vi "TrioMotion_Test.vi"() -> ()   [LabVIEW 2020]
panel:
  out "Error Out":errorcluster
  in  "stop":bool
  in  "Set Parameters":bool
  out "CommPort":fxp<+,3,3>
  in  "Open/ Close":bool
  in  "Connection":string(combo)
  out "IsOpen":bool
  in  "Error In (no error)":errorcluster
  in  "Connection":refnum<k7>(container)
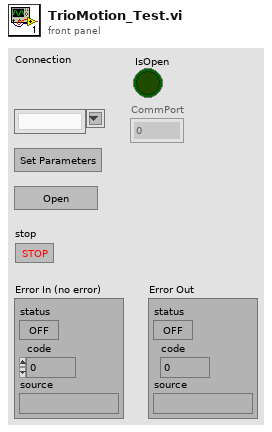
[diagram p1: front panel]
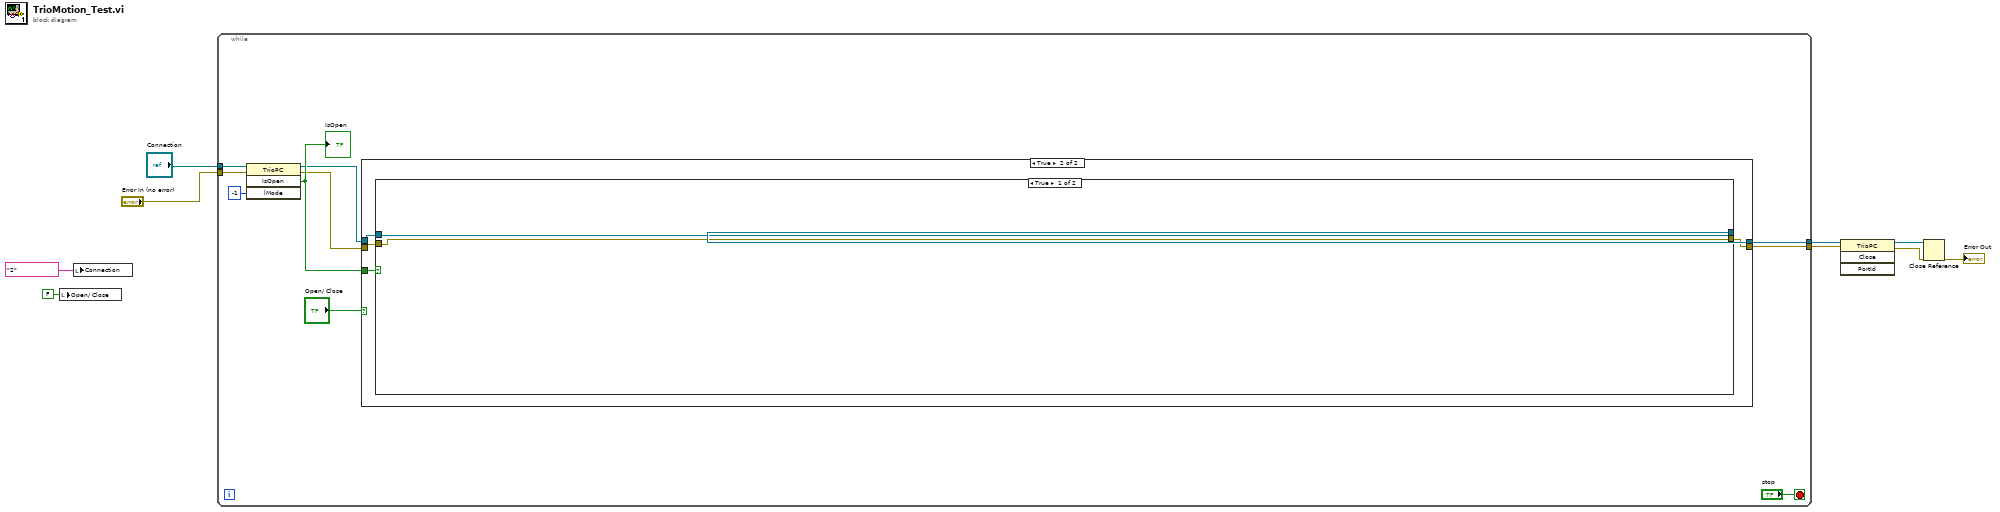
[diagram p0: block diagram]
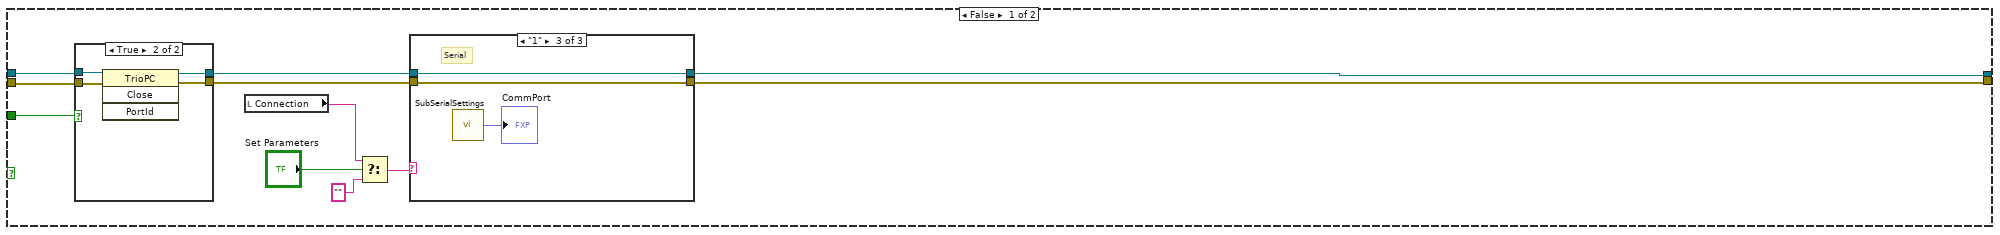
[diagram p2: hidden frame]
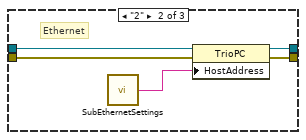
[diagram p4: hidden frame]
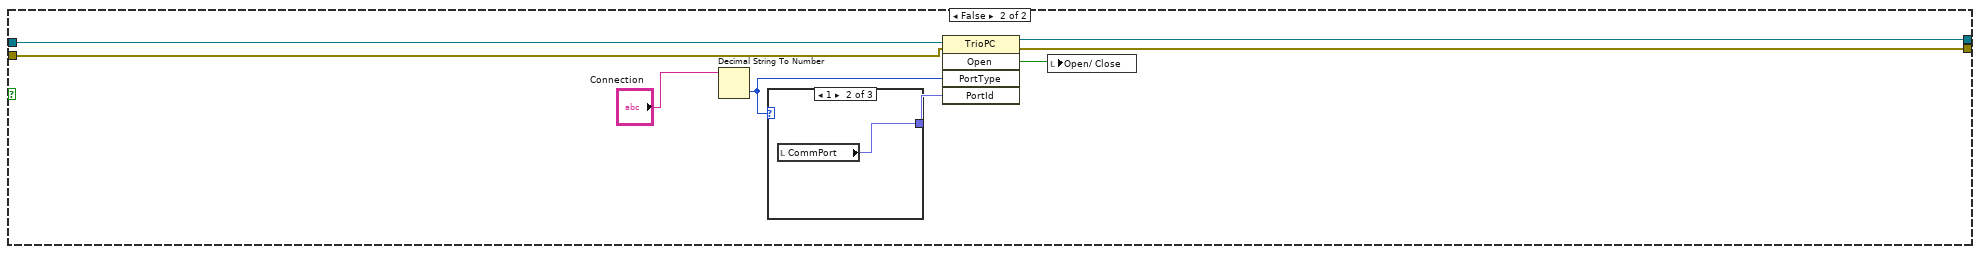
[diagram p6: hidden frame]
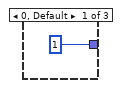
[diagram p7: hidden frame]
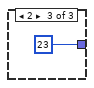
[diagram p8: hidden frame]
diagram:
  n1 = local write "Open/ Close"(FALSE ("Open/ Close")) -> ()
  n2 = local write "Connection"("2" ("Connection")) -> ()
  n3 = while {
    tunnel: "Connection" -> [w19]
    tunnel: "Error In (no error)" -> [w18]
    tunnel: [w11] -> w5
    tunnel: [w10] -> w4
    stop <- "stop" stop-if-true
    n4 = invoke class="TrioPC" method="IsOpen"(reference=w19, error in=w18, "lMode"=-1) -> (reference out=w14:refnum<k7>, error out=w13:errorcluster, "IsOpen"=w16:bool)  [unwired: 1 in, 1 out]
    "IsOpen" <- w16
    n5 = case shown="True" "Open/ Close" {
      tunnel: w14 -> [w30 w49]
      tunnel: w13 -> [w29 w48]
      tunnel: [w22 w51] -> w11
      tunnel: [w21 w50] -> w10
      tunnel: w16 -> [w28 w47]
      frame False {
        n6 = case shown="True" w28 {
          tunnel: w30 -> [w42 w46]
          tunnel: w29 -> [w41 w45]
          tunnel: [w42 w44] -> w24
          tunnel: [w41 w43] -> w23
          frame False {
          }
          frame True {
            n7 = invoke class="TrioPC" method="Close"(reference=w46, error in=w45) -> (reference out=w44:refnum<k7>, error out=w43:errorcluster)  [unwired: 2 in, 2 out]
          }
        }
        n8 = local read "Connection"() -> (w20:string)
        n9 = Select(t=w20, s="Set Parameters", f="") -> (s? t:f=w25:string)
        n10 = case shown="\"1\"" w25 {
          tunnel: w24 -> [w32 w35 w40]
          tunnel: w23 -> [w31 w34 w39]
          tunnel: [w32 w37 w40] -> w22
          tunnel: [w31 w36 w39] -> w21
          frame "", Default {
          }
          frame "2" {
            # "Ethernet"
            n11 = call "SubEthernetSettings.vi"() -> ("Ethernet IP Address 2"=w33:string)
            n12 = property class="TrioPC"(reference=w35, error in=w34, "HostAddress"=w33) -> (reference out=w37:refnum<k7>, error out=w36:errorcluster)
          }
          frame "1" {
            # "Serial"
            n13 = call "SubSerialSettings.vi"() -> ("CommPort"=→"CommPort":fxp<+,3,3>)
          }
        }
      }
      frame True {
        n14 = case shown="True" w47 {
          tunnel: w49 -> [w53 w59]
          tunnel: w48 -> [w52 w58]
          tunnel: [w53 w57] -> w51
          tunnel: [w52 w56] -> w50
          frame True {
          }
          frame False {
            n15 = Decimal String To Number(string="Connection") -> (number=w60:i32)  [unwired: 2 in, 1 out]
            n16 = case shown="1" w60 {
              tunnel: [i16 1 ("PortId") w63 i16 23 ("PortId")] -> w61
              frame 0, Default {
              }
              frame 1 {
                n17 = local read "CommPort"() -> (w63:fxp<+,3,3>)
              }
              frame 2 {
              }
            }
            n18 = invoke class="TrioPC" method="Open"(reference=w59, error in=w58, "PortType"=w60, "PortId"=w61) -> (reference out=w57:refnum<k7>, error out=w56:errorcluster, "Open"=w54:bool)  [unwired: 1 in, 2 out]
            n19 = local write "Open/ Close"(w54) -> ()
          }
        }
      }
    }
  }
  n20 = invoke class="TrioPC" method="Close"(reference=w5, error in=w4) -> (reference out=w3:refnum<k7>, error out=w2:errorcluster)  [unwired: 2 in, 2 out]
  n21 = Close Reference(reference=w3, error in (no error)=w2) -> (error out=→"Error Out":errorcluster)
